vi "color-picker.vi"(6 "VI Position":cluster{"Left":i16, "Top":i16}={"Left"=-1, "Top"=-1}, 11 "input":u32(colorbox)) -> (2 "accepted?":bool, 3 "Resolved Color":u32(colorbox))   [LabVIEW 2021]
uses:
  <vilib>/Utility/miscctls.llb/LVRectTypeDef.ctl
panel:
  in  "cancel":bool
  in  "ok":bool
  in  "B-selector":u8
  in  "G-selector":u8
  in  "R-selector":u8
  in  "B-number":u8(slide) scale=0.0..255.0
  out "B":u32[](array[colorbox])
  in  "G-number":u8(slide) scale=0.0..255.0
  out "G":u32[](array[colorbox])
  in  "R-number":u8(slide) scale=0.0..255.0
  out "R":u32[](array[colorbox])
  in  "Hex Color":u32 format="%06x"
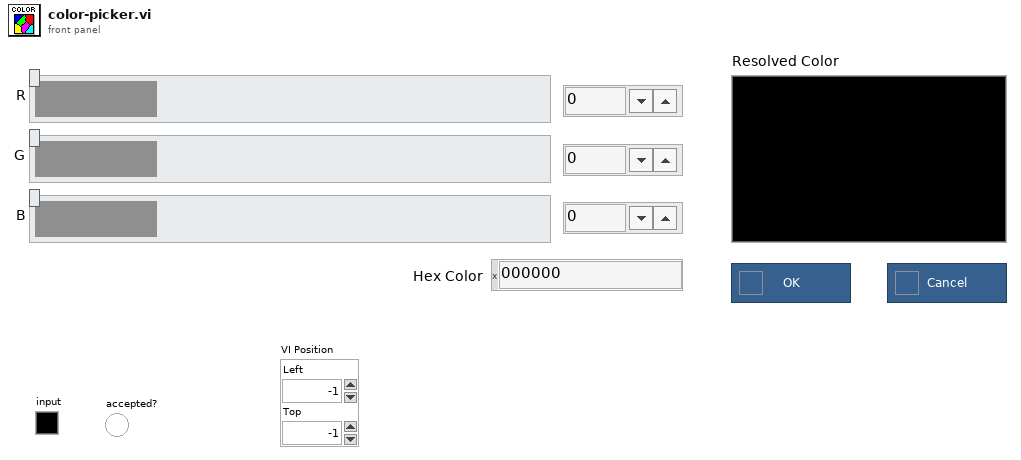
[diagram p1: front panel]
types:
  T1 = typedef "LVRectTypeDef.ctl" = cluster{"Left":i16, "Top":i16, "Right":i16, "Bottom":i16}
  T2 = typedef "LVPointTypeDef.ctl" = cluster{"Horizontal":i16, "Vertical":i16}
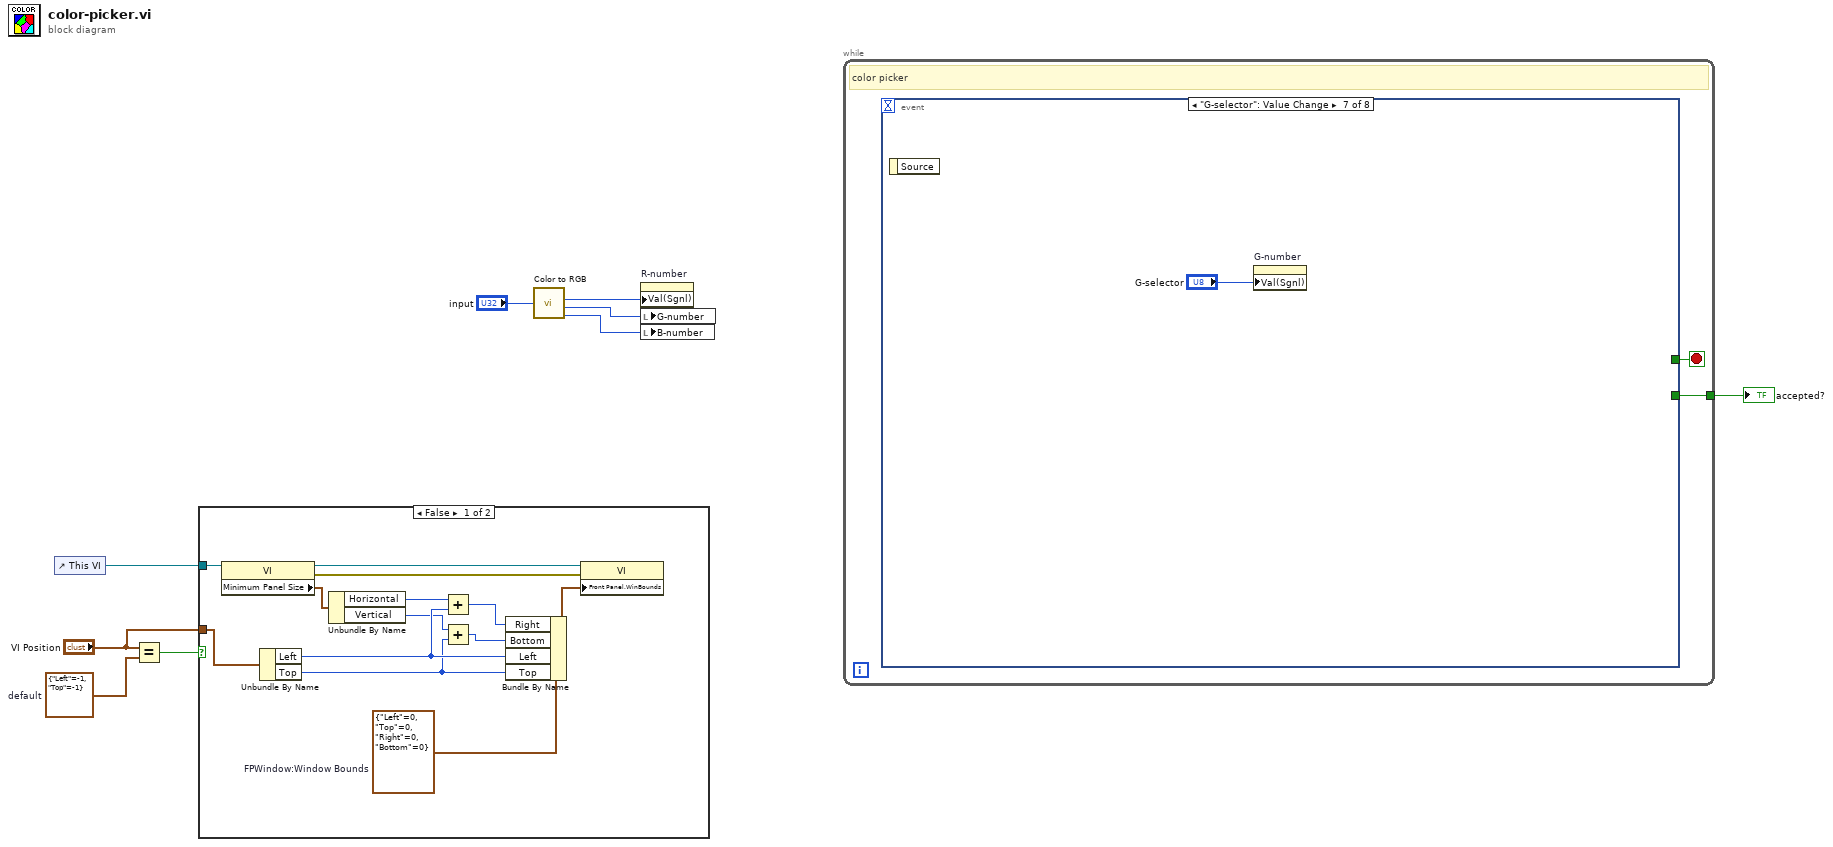
[diagram p0: block diagram]
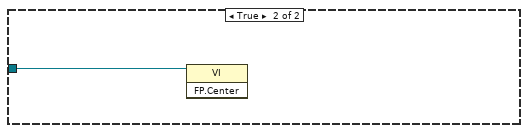
[diagram p2: hidden frame]
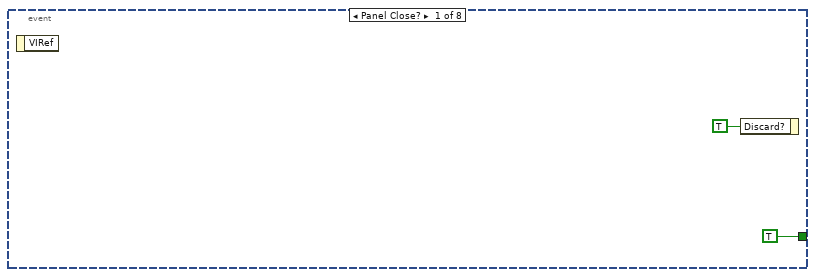
[diagram p3: hidden frame]
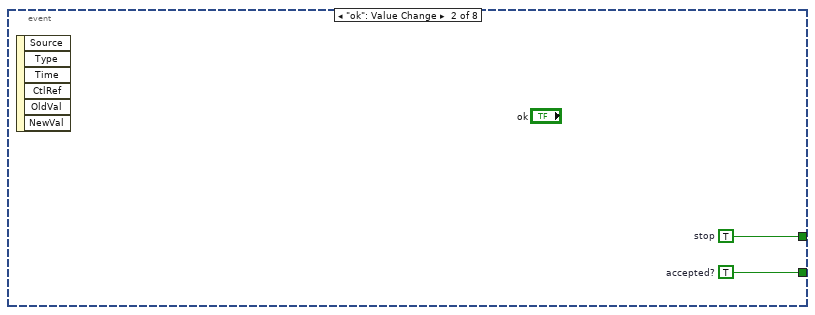
[diagram p4: hidden frame]
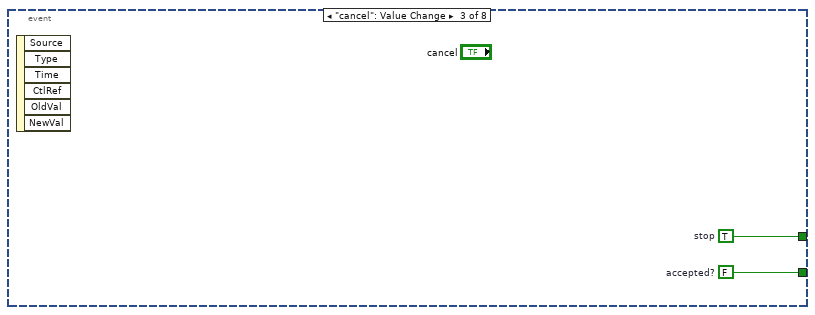
[diagram p5: hidden frame]
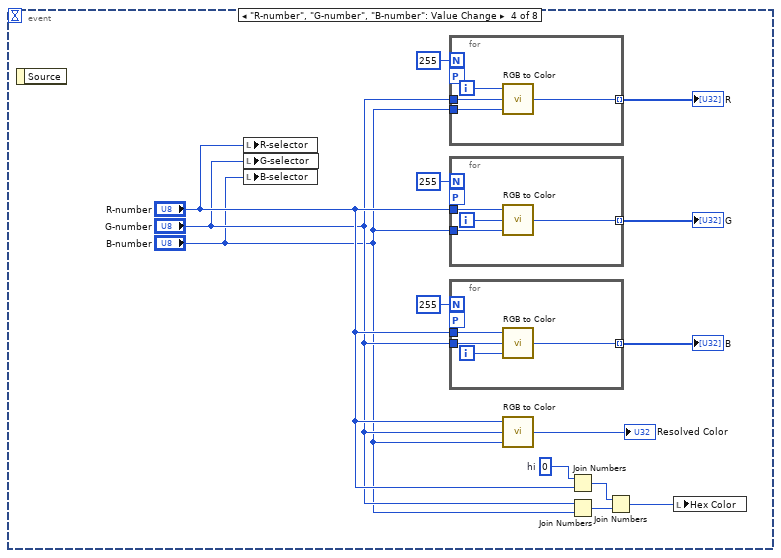
[diagram p6: hidden frame]
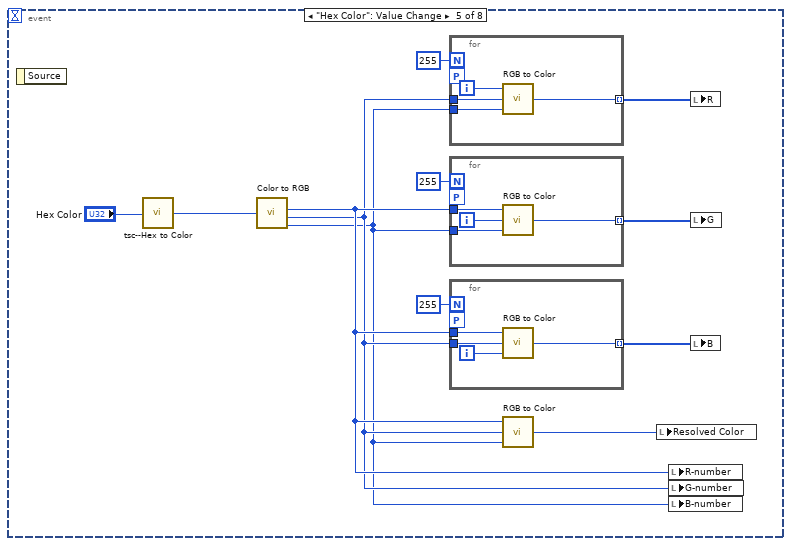
[diagram p7: hidden frame]
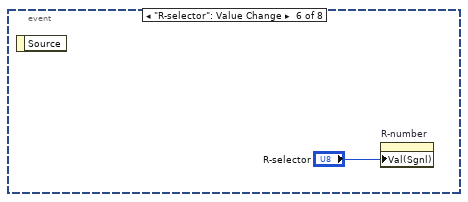
[diagram p8: hidden frame]
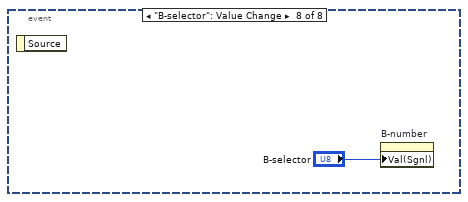
[diagram p9: hidden frame]
diagram:
  w3 = cluster{"Left":i16, "Top":i16} {"Left"=-1, "Top"=-1}  # default
  n1 = control-ref of="This VI"() -> (w4:refnum<vi>)
  n2 = Equal?(x="VI Position", y=w3) -> (x = y?=w2:bool)
  n3 = case shown="False" w2 {
    tunnel: w4 -> [w22 w23]
    tunnel: "VI Position" -> [w18 _]
    frame False {
      w17 = T1 {"Left"=0, "Top"=0, "Right"=0, "Bottom"=0}  # FPWindow:Window Bounds
      n4 = property class="VI"(reference=w22) -> (reference out=w21:refnum<vi>, error out=w20:errorcluster, "Minimum Panel Size"=w19:T2)  [unwired: 1 in]
      n5 = Unbundle By Name(w18) -> ("Left"=w16:i16, "Top"=w11:i16)
      n6 = Unbundle By Name(w19) -> ("Horizontal"=w15:i16, "Vertical"=w12:i16)
      n7 = Add(x=w15, y=w16) -> (x+y=w14:i16)
      n8 = Add(x=w12, y=w11) -> (x+y=w10:i16)
      n9 = Bundle By Name(cluster=w17, "Right"=w14, "Bottom"=w10, "Left"=w16, "Top"=w11) -> (w13:T1)
      n10 = property class="VI"(reference=w21, error in=w20, "Front Panel.WinBounds"=w13) -> ()  [unwired: 2 out]
    }
    frame True {
      n11 = invoke class="VI" method="FP.Center"(reference=w23) -> ()  [unwired: 2 in, 3 out]
    }
  }
  n12 = call <vilib>:"Color to RGB.vi"("Color"="input") -> ("R"=w8:u8, "G"=w7:u8, "B"=w6:u8)  [unwired: 1 out]
  n13 = property on="R-number" class="Slide (strict)"("Val(Sgnl)"=w8) -> ()  [unwired: 2 in, 2 out]
  n14 = local write "G-number"(w7) -> ()
  n15 = local write "B-number"(w6) -> ()
  n16 = while {
    tunnel: [w24] -> w5
    stop <- w25 stop-if-true
    # "color picker"
    n17 = event shown="[6] \"G-selector\": Value Change" {
      selector: _ -> [_ _ _ _ _ _ _ _]
      dyn-events: _ -> [_ _ _ _ _ _ _ _]
      timeout: _ -> [_ _ _ _ _ _ _ _]
      tunnel: [TRUE w29 w31 _ _ _ _ _] -> w25
      tunnel: [_ w28 w30 _ _ _ _ _] -> w24
      event Panel Close? {
        n18 = event-data() -> ()  [unwired: 1 in, 1 out]
        n19 = event-data("Discard?"=TRUE) -> ()  [unwired: 1 in, 1 out]
      }
      event "ok": Value Change {
        w28 = TRUE  # accepted?
        w29 = TRUE  # stop
        n20 = event-data() -> ()  [unwired: 1 in, 6 out]
      }
      event "cancel": Value Change {
        w30 = FALSE  # accepted?
        w31 = TRUE  # stop
        n21 = event-data() -> ()  [unwired: 1 in, 6 out]
      }
      event "R-number", "G-number", "B-number": Value Change {
        w39 = u8 0  # hi
        n22 = event-data() -> ()  [unwired: 1 in, 1 out]
        n23 = local write "R-selector"("R-number") -> ()
        n24 = local write "G-selector"("G-number") -> ()
        n25 = local write "B-selector"("B-number") -> ()
        n26 = for {
          N: 255 -> [_]
          tunnel: "G-number" -> [w57]
          tunnel: "B-number" -> [w56]
          tunnel: [w54] -> w44 mode=indexing
          workers-P: _ -> [_]
          i -> [w55]
          n27 = call <vilib>:"RGB to Color.vi"("B"=w56, "G"=w57, "R"=w55) -> ("Color"=w54:u32)
        }
        "R" <- w44
        n28 = for {
          N: 255 -> [_]
          tunnel: "B-number" -> [w53]
          tunnel: [w52] -> w41 mode=indexing
          tunnel: "R-number" -> [w50]
          workers-P: _ -> [_]
          i -> [w51]
          n29 = call <vilib>:"RGB to Color.vi"("B"=w53, "G"=w51, "R"=w50) -> ("Color"=w52:u32)
        }
        "G" <- w41
        n30 = for {
          N: 255 -> [_]
          tunnel: "R-number" -> [w47]
          tunnel: [w49] -> w40 mode=indexing
          tunnel: "G-number" -> [w46]
          workers-P: _ -> [_]
          i -> [w48]
          n31 = call <vilib>:"RGB to Color.vi"("B"=w48, "G"=w46, "R"=w47) -> ("Color"=w49:u32)
        }
        "B" <- w40
        n32 = call <vilib>:"RGB to Color.vi"("B"="B-number", "G"="G-number", "R"="R-number") -> ("Color"=→"Resolved Color":u32)
        n33 = Join Numbers(hi=w39, lo="R-number") -> ((hi.lo)=w37:u16)
        n34 = Join Numbers(hi="G-number", lo="B-number") -> ((hi.lo)=w38:u16)
        n35 = Join Numbers(hi=w37, lo=w38) -> ((hi.lo)=w36:u32)
        n36 = local write "Hex Color"(w36) -> ()
      }
      event "Hex Color": Value Change {
        n37 = event-data() -> ()  [unwired: 1 in, 1 out]
        n38 = call "tsc--Hex to Color.vi"("Hex String"="Hex Color") -> ("Color Box"=w65:u32)  [unwired: 4 in]
        n39 = call <vilib>:"Color to RGB.vi"("Color"=w65) -> ("R"=w60:u8, "G"=w59:u8, "B"=w58:u8)  [unwired: 1 out]
        n40 = for {
          N: 255 -> [_]
          tunnel: w59 -> [w81]
          tunnel: w58 -> [w80]
          tunnel: [w78] -> w64 mode=indexing
          workers-P: _ -> [_]
          i -> [w79]
          n41 = call <vilib>:"RGB to Color.vi"("B"=w80, "G"=w81, "R"=w79) -> ("Color"=w78:u32)
        }
        n42 = for {
          N: 255 -> [_]
          tunnel: w58 -> [w77]
          tunnel: [w76] -> w63 mode=indexing
          tunnel: w60 -> [w74]
          workers-P: _ -> [_]
          i -> [w75]
          n43 = call <vilib>:"RGB to Color.vi"("B"=w77, "G"=w75, "R"=w74) -> ("Color"=w76:u32)
        }
        n44 = for {
          N: 255 -> [_]
          tunnel: w60 -> [w71]
          tunnel: [w73] -> w62 mode=indexing
          tunnel: w59 -> [w70]
          workers-P: _ -> [_]
          i -> [w72]
          n45 = call <vilib>:"RGB to Color.vi"("B"=w72, "G"=w70, "R"=w71) -> ("Color"=w73:u32)
        }
        n46 = call <vilib>:"RGB to Color.vi"("B"=w58, "G"=w59, "R"=w60) -> ("Color"=w61:u32)
        n47 = local write "Resolved Color"(w61) -> ()
        n48 = local write "R-number"(w60) -> ()
        n49 = local write "G-number"(w59) -> ()
        n50 = local write "B-number"(w58) -> ()
        n51 = local write "R"(w64) -> ()
        n52 = local write "G"(w63) -> ()
        n53 = local write "B"(w62) -> ()
      }
      event "R-selector": Value Change {
        n54 = event-data() -> ()  [unwired: 1 in, 1 out]
        n55 = property on="R-number" class="Slide (strict)"("Val(Sgnl)"="R-selector") -> ()  [unwired: 2 in, 2 out]
      }
      event "G-selector": Value Change {
        n56 = event-data() -> ()  [unwired: 1 in, 1 out]
        n57 = property on="G-number" class="Slide (strict)"("Val(Sgnl)"="G-selector") -> ()  [unwired: 2 in, 2 out]
      }
      event "B-selector": Value Change {
        n58 = event-data() -> ()  [unwired: 1 in, 1 out]
        n59 = property on="B-number" class="Slide (strict)"("Val(Sgnl)"="B-selector") -> ()  [unwired: 2 in, 2 out]
      }
    }
  }
  "accepted?" <- w5
